vi "Panel Init Flow Meter.vi"(0 "Com Flow Computer":refnum<visa-resource-name>="COM1", 11 "Error In":errorcluster) -> (4 "Use Dry Gas Meter Out?":bool=TRUE, 6 "Use GasFlow Computer Out?":bool=TRUE, 8 "Baro,BTUF,u,Z,T":string[][](array[string]), 15 "Error Out":errorcluster)   [LabVIEW 2009]
uses:
  SL9200 Flow Calc/SL9200_Registers.ctl
panel:
  in  "Gas Pressure":string="7.5"
  in  "Gas Temperature":string="78"
  in  "Use Dry Gas Meter?":bool=TRUE
  out "Array":string[](array[string])
  in  "Barometric (inHg)":string="29.5"
  in  "Flow Z":string="1"
  in  "stop":bool
  in  "Use GasFlow Computer?":bool
  in  "BTU per Ft3":string="990"
  in  "Density (LB/FT3)":string=".051"
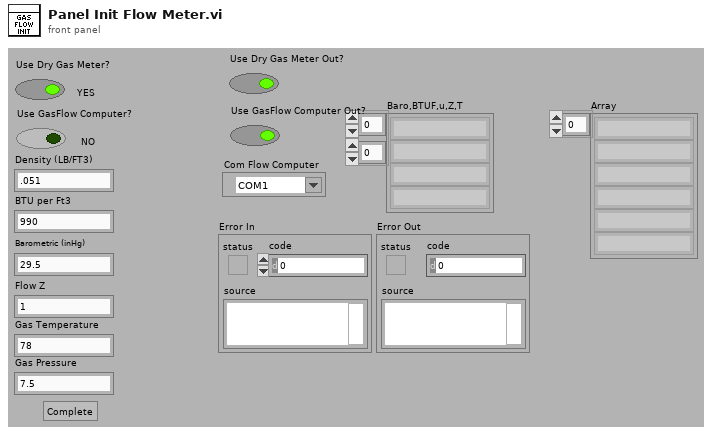
[diagram p1: front panel]
types:
  T1 = typedef "SL9200_Registers.ctl" = u8
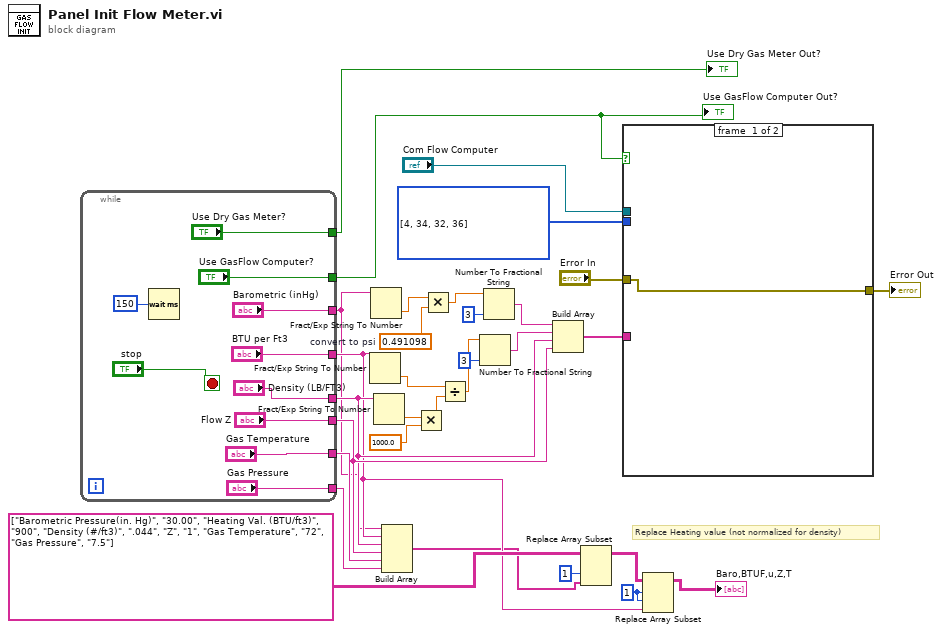
[diagram p0: block diagram]
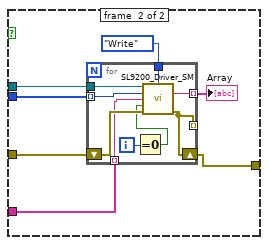
[diagram p2: hidden frame]
diagram:
  w8 = 1 ("index (row)")
  w17 = 0.491098  # convert to psi
  w30 = T1[] [4, 34, 32, 36] items=["Heat_Flow", "Mass_Flow", "Corrected_Volume_Flow", "Volume_Flow", "Temperature", "Temperature2", "Delta_Temperature", "Pressure", "Diff_Pressure", "Density", "Spec_Enthalpy", "Date", "Time", "Level", "Peak_Demand", "Demand_Last_Hour", "Peak_Demand_Time", "Peak_Demand_Date", "Viscosity", "Reynolds_Number", "Heat_Total", "Grand_Heat_Total", "Mass_Total", "Grand_Mass", "Corrected_Volume_Total", "Grand_Corrected_Volume", "Volume_Total", "Grand_Volume", "Totalizer_Reset", "Alarm_Reset", "Barometric", "Fluid_Type", "Reference_Density", "Therm_Expansion_Coef", "Combustion_Heat", "Specific_Heat", "Flow_Z_Factor", "Ref_Z_Factor", "Isentropic_Exponent", "Viscosity_A", "Viscosity_B", "Reference_Temperature", "Calibration_Density", "Base_Density_H2O_4C", "Per_Mole_N2", "Per_Mole_CO2", "Tag_Number", "Software_Version", "Hardware_Version", "Order_Code", "Serial_Number", "Sensor_Serial_Num"]
  # "Replace Heating value (not normalized for density)"
  n1 = while {
    tunnel: ["Barometric (inHg)"] -> w2
    tunnel: ["BTU per Ft3"] -> w3
    tunnel: ["Flow Z"] -> w5
    tunnel: ["Density (LB/FT3)"] -> w4
    tunnel: ["Use GasFlow Computer?"] -> w15
    tunnel: ["Use Dry Gas Meter?"] -> w14
    tunnel: ["Gas Temperature"] -> w6
    tunnel: ["Gas Pressure"] -> w7
    stop <- "stop" stop-if-true
    n2 = Wait (ms)(milliseconds to wait=u32 150) -> ()  [unwired: 1 out]
  }
  "Use GasFlow Computer Out?" <- w15
  "Use Dry Gas Meter Out?" <- w14
  n3 = Fract/Exp String To Number(string=w3) -> (number=w24:dbl)  [unwired: 3 in, 1 out]
  n4 = Fract/Exp String To Number(string=w2) -> (number=w18:dbl)  [unwired: 3 in, 1 out]
  n5 = Fract/Exp String To Number(string=w4) -> (number=w27:dbl)  [unwired: 3 in, 1 out]
  n6 = Build Array(w2, w3, w4, w5, w6, w7) -> (w1:string[])
  n7 = Multiply(x=w27, y=1000.0) -> (x*y=w25:dbl)
  n8 = Multiply(x=w18, y=w17) -> (x*y=w19:dbl)
  n9 = Divide(x=w24, y=w25) -> (x/y=w23:dbl)
  n10 = Number To Fractional String(number=w23, precision (6)=i16 3) -> (F-format string=w22:string)  [unwired: 2 in]
  n11 = Number To Fractional String(number=w19, precision (6)=i16 3) -> (F-format string=w16:string)  [unwired: 2 in]
  n12 = Build Array(w16, w22, w4, w5) -> (w11:string[])
  n13 = Replace Array Subset(array=string[][] [["Barometric Pressure(in. Hg)", "30.00"], ["Heating Val. (BTU/ft3)", "900"], ["Density (#/ft3)", ".044"], ["Z", "1"], ["Gas Temperature", "72"], ["Gas Pressure", "7.5"]] ("appended array"), new element=w1, index (col)=1 ("disabled index (col)")) -> (w10:string[][])  [unwired: 1 in]
  n14 = case shown="True" w15 {
    tunnel: "Com Flow Computer" -> [_ w49]
    tunnel: w30 -> [_ w47]
    tunnel: "Error In" -> [w42 w46]
    tunnel: [w42 w45] -> w28
    tunnel: w11 -> [_ w44]
    frame #0 {
    }
    frame #1 {
      n15 = for {
        tunnel: w49 -> [w58]
        tunnel: [w57] -> w43 mode=indexing
        tunnel: w47 -> [w54] mode=indexing
        shift-right: [w51] -> w45
        shift-left: w46 -> [w56]
        tunnel: enum16{"Read", "Write"}."Write" ("Mode") -> [w55]
        tunnel: w44 -> [w53] mode=indexing
        tunnel: [w51] -> _ mode=indexing
        i -> [w52]
        n16 = Equal To 0?(x=w52) -> (x = 0?=w50:bool)
        n17 = call "SL9200_Driver_SM.vi"("ComPort"=w58, "Mode"=w55, "Register"=w54, "Write Data"=w53, "InitSerial?"=w50, "Error In"=w56) -> ("Response"=w57:string, "Error Out"=w51:errorcluster)  [unwired: 7 in, 1 out]
      }
      "Array" <- w43
    }
  }
  "Error Out" <- w28
  n18 = Replace Array Subset(array=w10, new element=w3, index (row)=w8, index (col)=w8) -> (→"Baro,BTUF,u,Z,T":string[][])
